vi "Zero.vi"(0 "object in":refnum<class "CoriFlowBFS1Plus.lvclass">, 5 "error in (no error)":errorcluster) -> (14 "object out":refnum<class "CoriFlowBFS1Plus.lvclass">, 19 "error out":errorcluster)   [LabVIEW 2021, in "CoriFlowBFS1Plus.lvclass"]
uses:
  CoriFlowBFS1Plus.lvclass
  CoriFlowBFS1Plus.lvclass/CoriFlowBFS1Plus.ctl
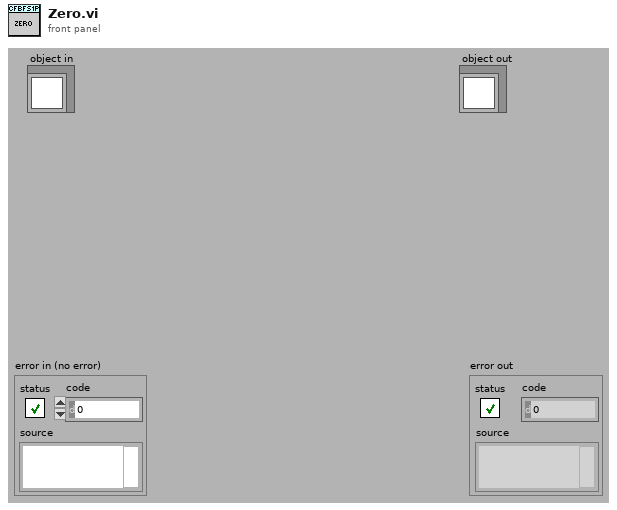
[diagram p1: front panel]
types:
  T1 = typedef "Z_BFS_type.ctl" = cluster{"VISA_Name":refnum<visa-resource-name>, "density_g_L":dbl, "Capacity":dbl, "Capacity units conversion":dbl}
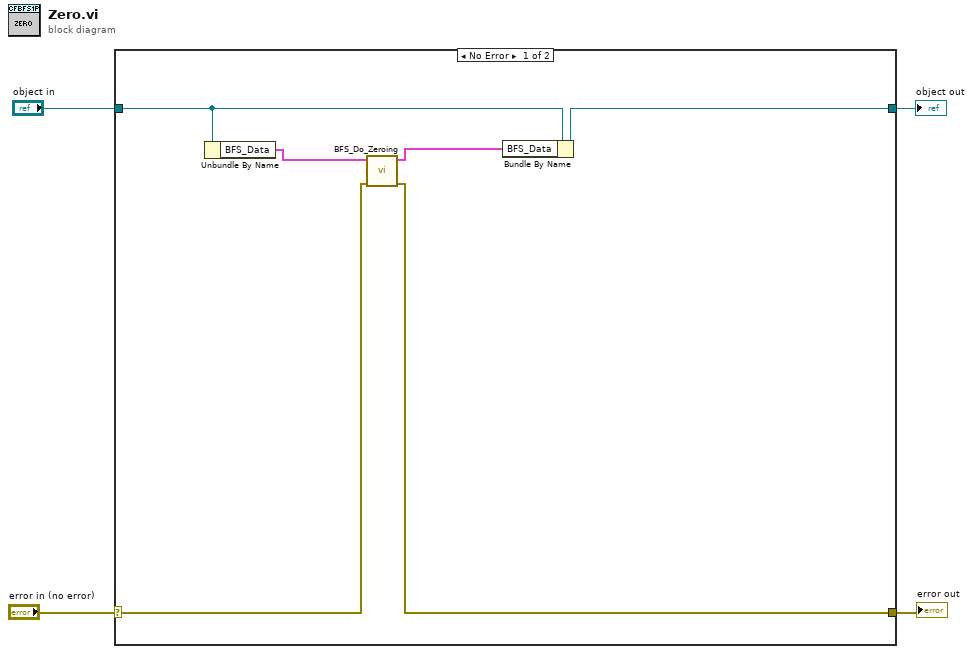
[diagram p0: block diagram]
diagram:
  n1 = case shown="No Error" "error in (no error)" {
    selector: "error in (no error)" -> [w6 w12]
    tunnel: [w5 w12] -> w3
    tunnel: [w9 w11] -> w1
    tunnel: "object in" -> [w10 w11]
    frame No Error {
      n2 = Unbundle By Name(w10) -> ("BFS_Data"=w8:T1)
      n3 = call "BFS_Do_Zeroing.vi"("error in"=w6, "BFS_type_In"=w8) -> ("error out"=w5:errorcluster, "BFS_type_Out"=w7:T1)  [unwired: 8 in]
      n4 = Bundle By Name(cluster=w10, "BFS_Data"=w7) -> (w9:refnum<class "CoriFlowBFS1Plus.lvclass">)
    }
    frame Error {
    }
  }
  "error out" <- w3
  "object out" <- w1
